vi "Examen 2 maquina de estados.vi"() -> ()   [LabVIEW 2021]
panel:
  out "LED":bool
  out "PUERTA":bool
  in  "Reset":bool
  out "#cafe":dbl
  in  "MANTENIMIENTO":bool
  out "#dulces":dbl
  out "#cafe 2":dbl
  out "#colombian":dbl
  out "#coca":dbl
  out "#pastel":dbl
  out "#dorito":dbl
  in  "Verificar":string
  in  "Coca-cola":bool
  in  "stop":bool
  out "Display":string
  out "CAMBIO":dbl
  out "EFECTIVO":dbl
  in  "COMPRAR":bool
  in  "capuchino":bool
  in  "coffe":bool
  in  "snacks Doritos":bool
  in  "Colombiana":bool
  in  "Candies":bool
  in  "pastel":bool
  in  "10":bool
  in  "20":bool
  # "MONEDAS"
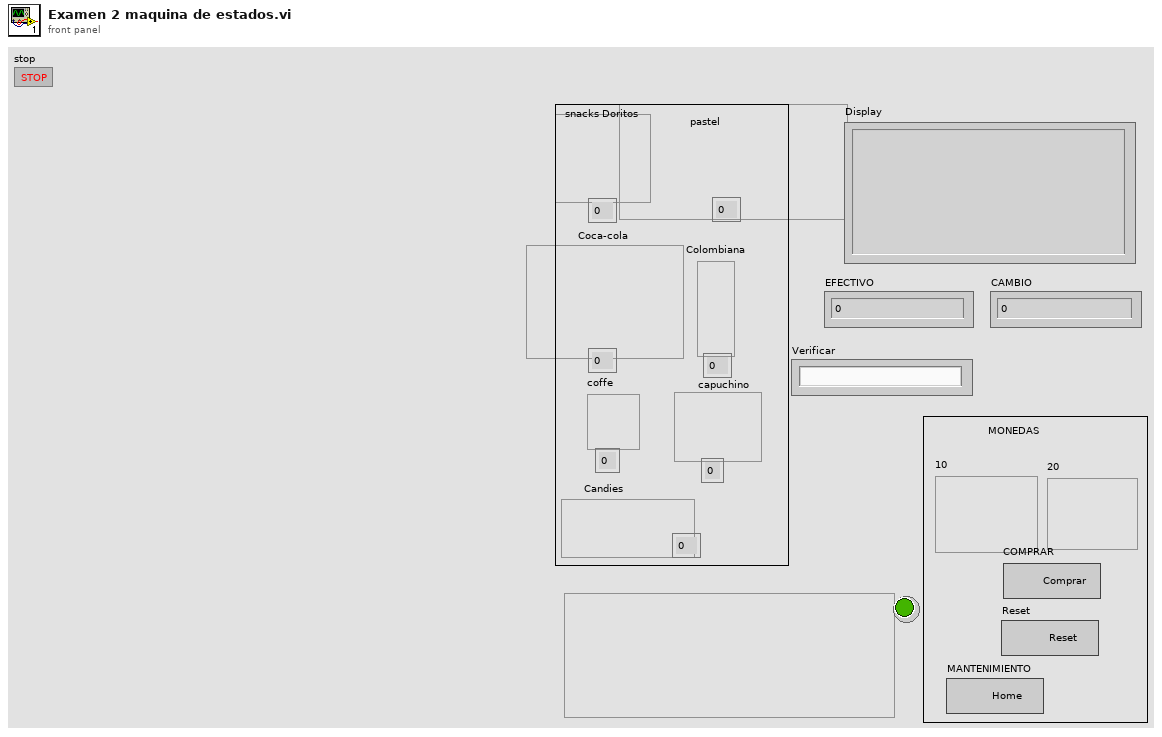
[diagram p1: front panel]
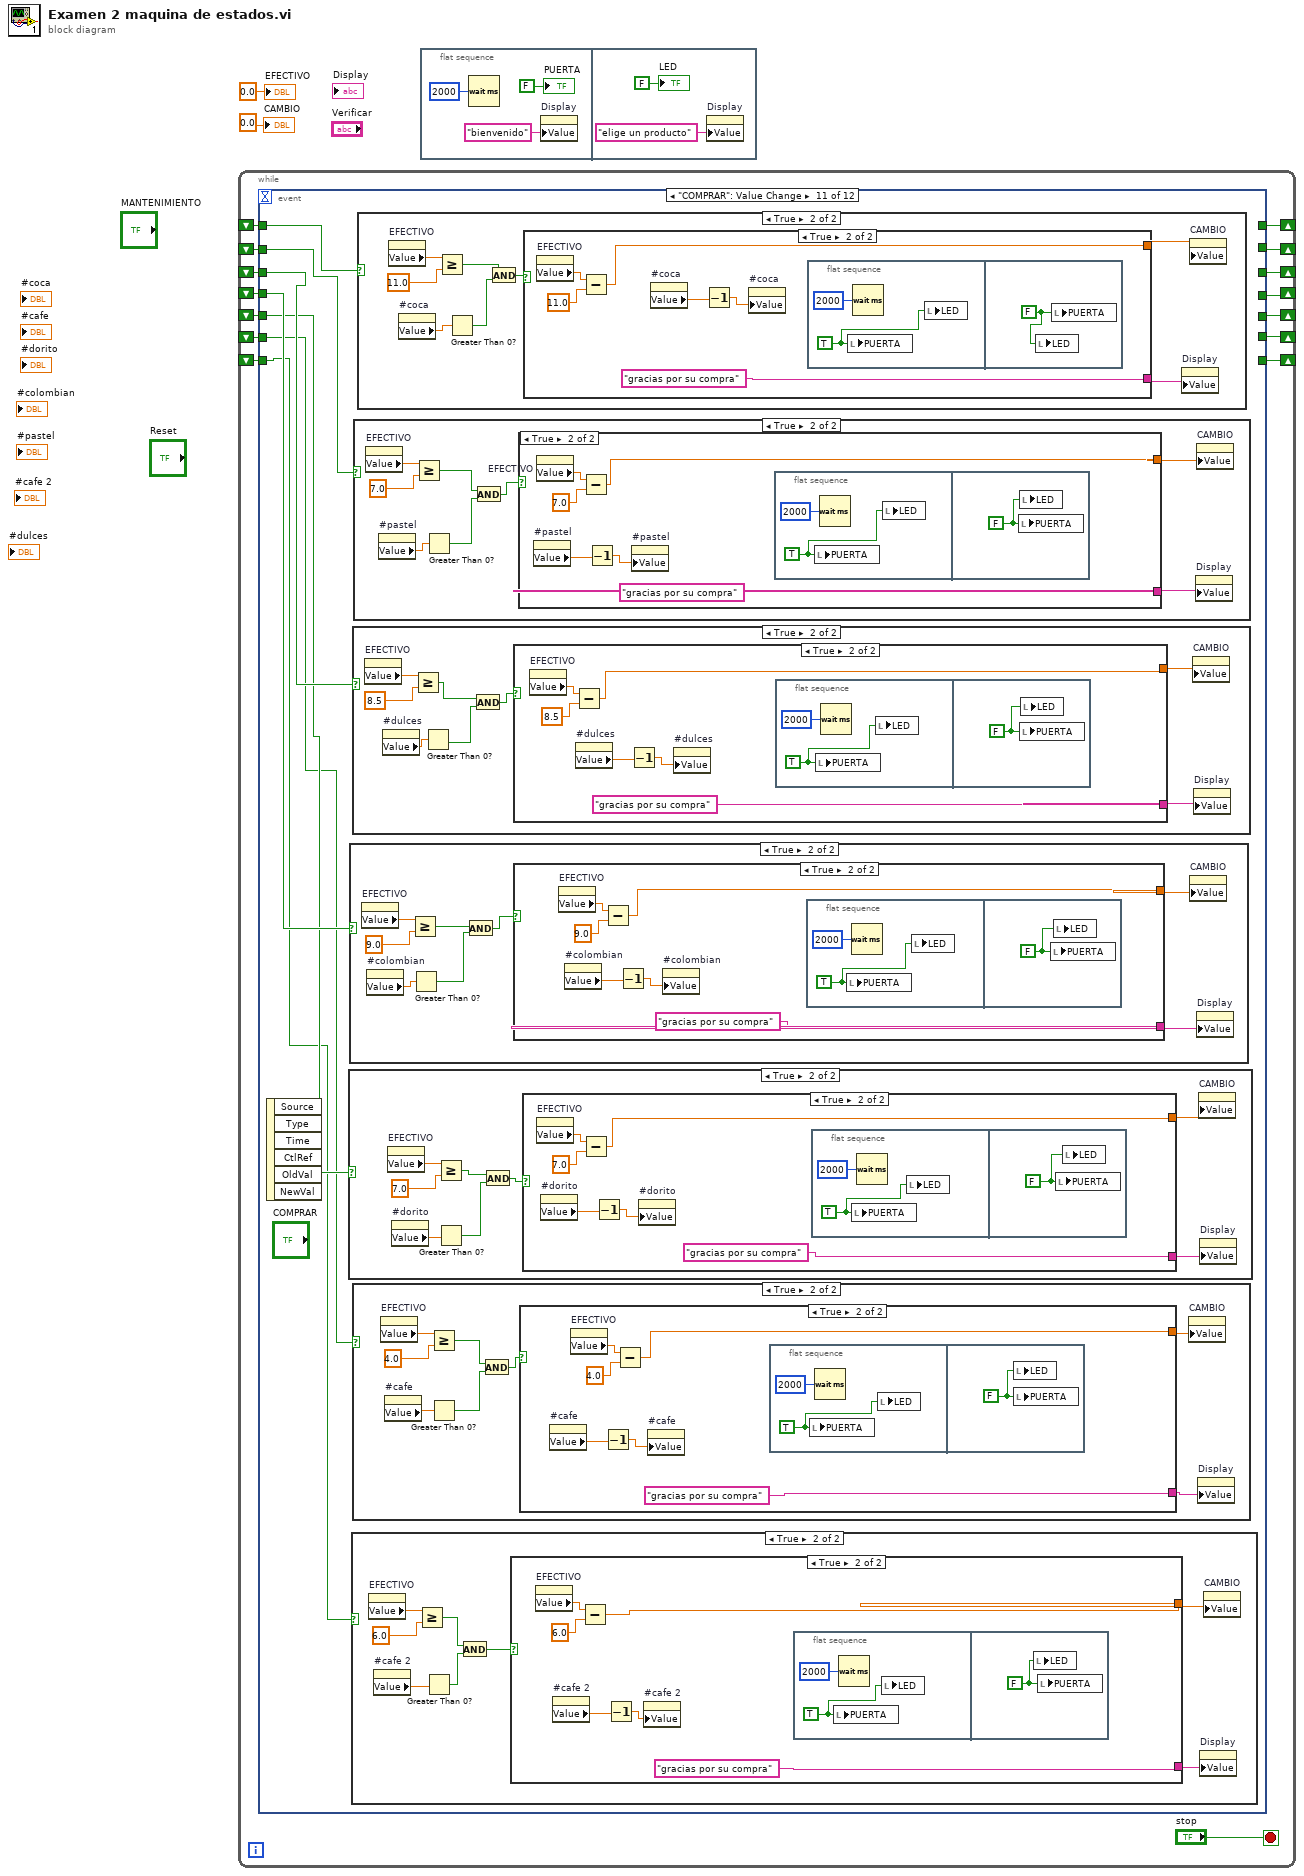
[diagram p0: block diagram]
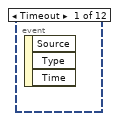
[diagram p2: hidden frame]
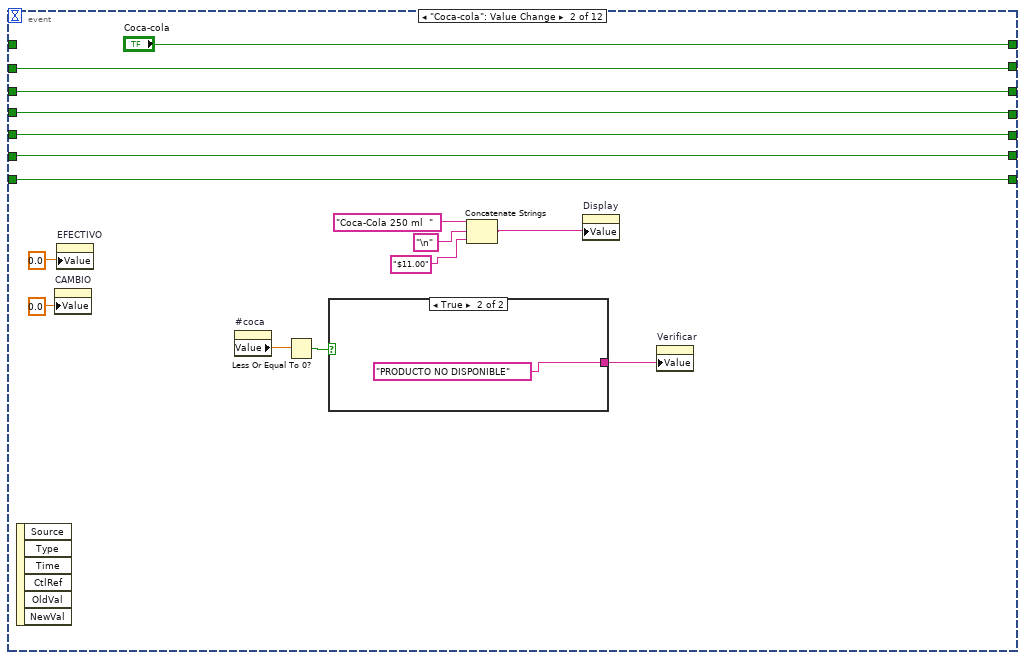
[diagram p3: hidden frame]
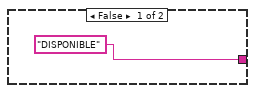
[diagram p4: hidden frame]
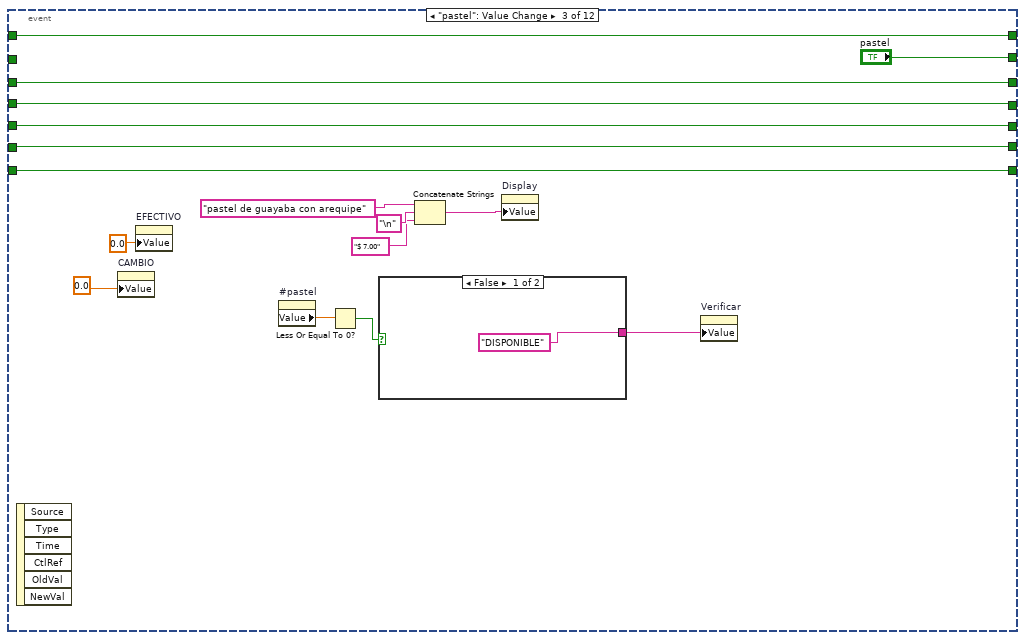
[diagram p5: hidden frame]
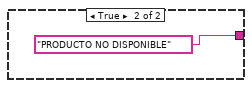
[diagram p6: hidden frame]
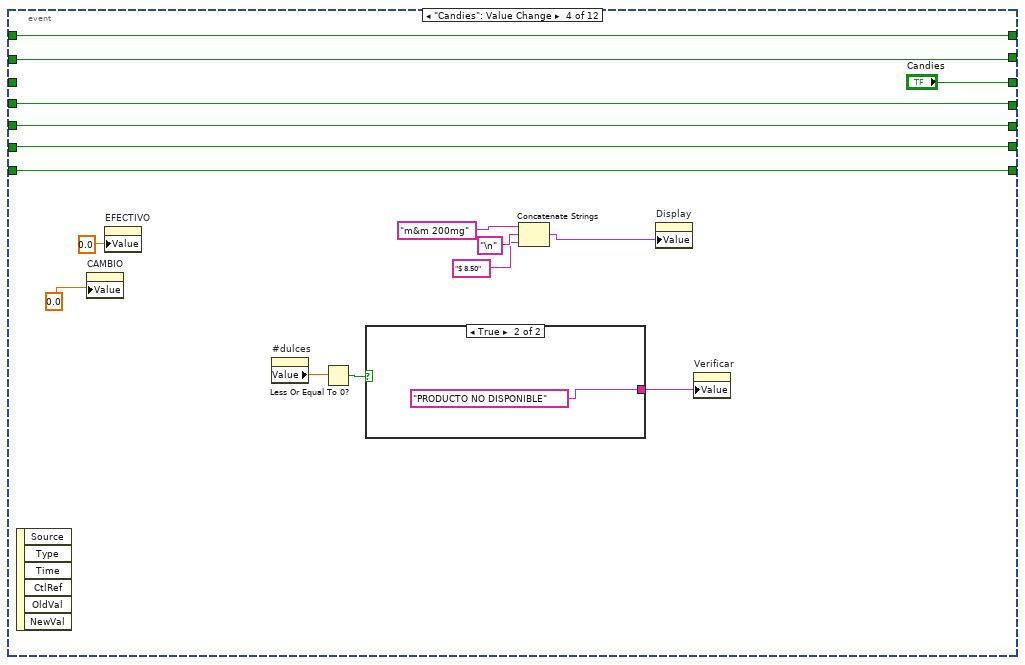
[diagram p7: hidden frame]
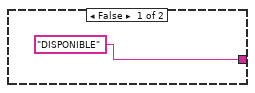
[diagram p8: hidden frame]
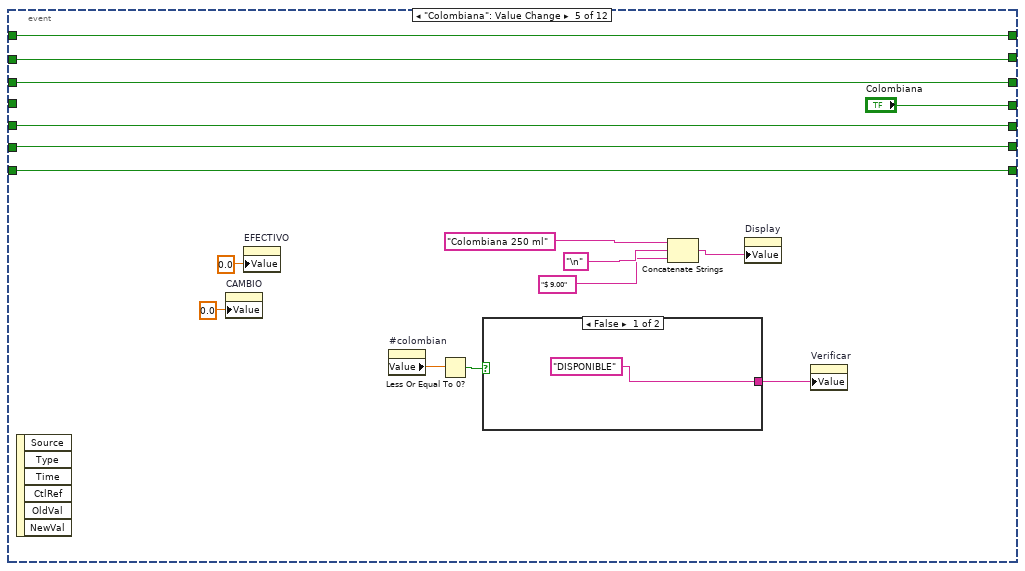
[diagram p9: hidden frame]
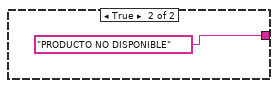
[diagram p10: hidden frame]
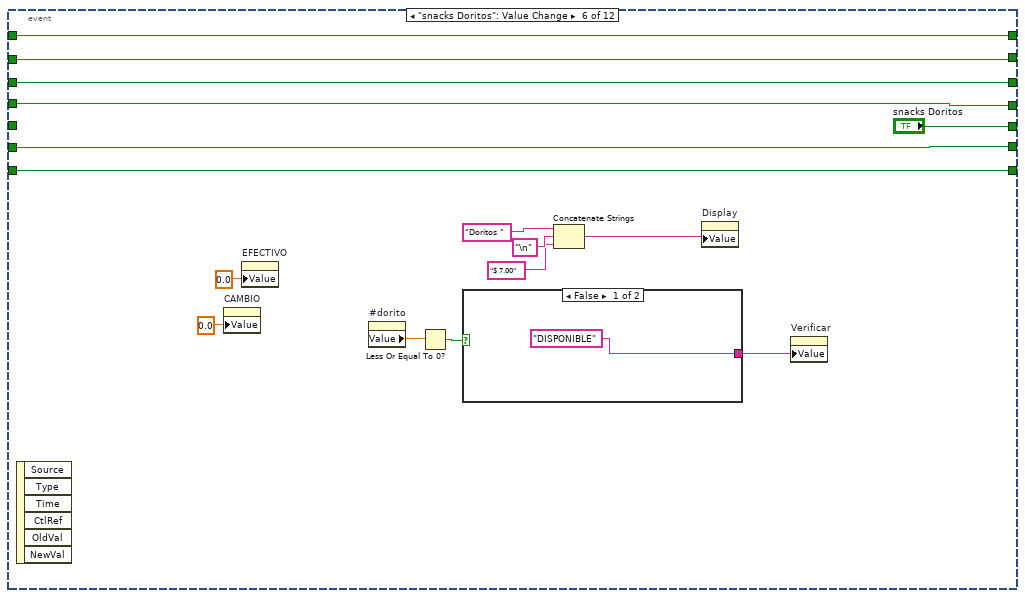
[diagram p11: hidden frame]
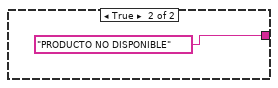
[diagram p12: hidden frame]
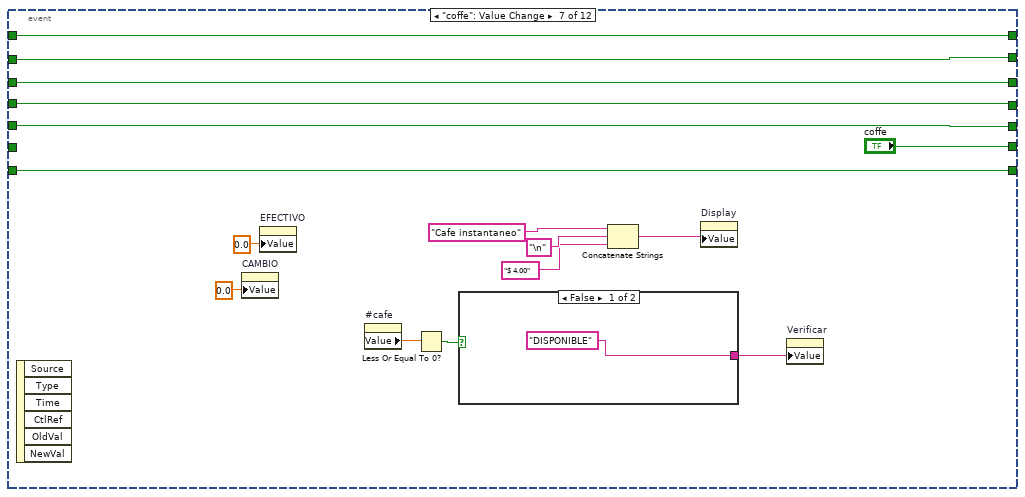
[diagram p13: hidden frame]
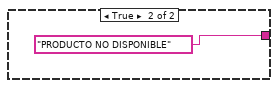
[diagram p14: hidden frame]
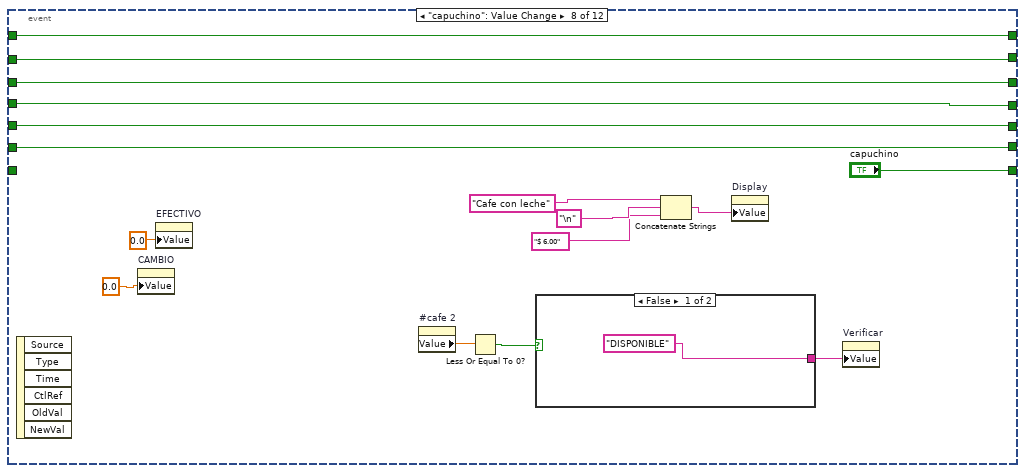
[diagram p15: hidden frame]
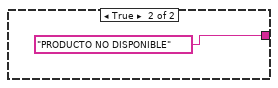
[diagram p16: hidden frame]
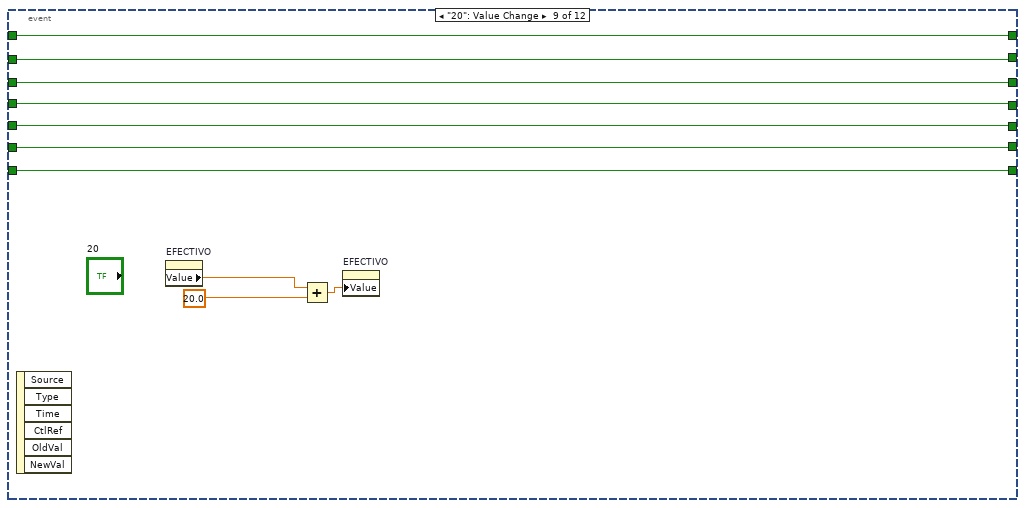
[diagram p17: hidden frame]
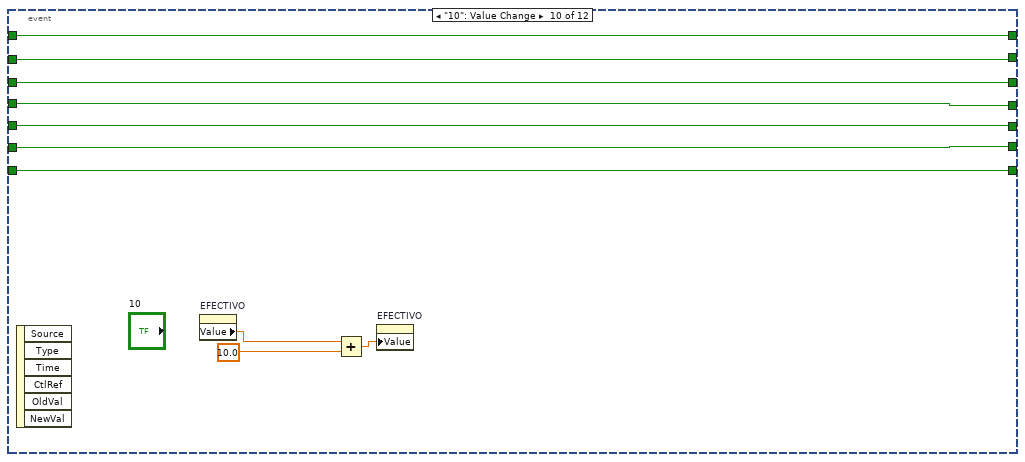
[diagram p18: hidden frame]
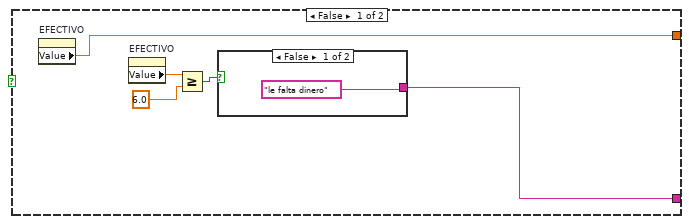
[diagram p20: hidden frame]
diagram:
  n1 = while {
    shift-right: [w16] -> _
    shift-left: _ -> [w15]
    shift-right: [w14] -> _
    shift-left: _ -> [w13]
    shift-right: [w12] -> _
    shift-left: _ -> [w11]
    shift-right: [w10] -> _
    shift-left: _ -> [w9]
    shift-right: [w8] -> _
    shift-left: _ -> [w7]
    shift-right: [w6] -> _
    shift-left: _ -> [w5]
    shift-right: [w4] -> _
    shift-left: _ -> [w3]
    stop <- "stop" stop-if-true
    n2 = event shown="[10] \"COMPRAR\": Value Change" {
      selector: _ -> [_ _ _ _ _ _ _ _ _ _ _ _]
      dyn-events: _ -> [_ _ _ _ _ _ _ _ _ _ _ _]
      timeout: _ -> [_ _ _ _ _ _ _ _ _ _ _ _]
      tunnel: [_ "Coca-cola" w51 w69 w87 w105 w123 w141 w150 w160 _ _] -> w16
      tunnel: w15 -> [_ _ w51 w69 w87 w105 w123 w141 w150 w160 w170 _]
      tunnel: [_ w30 "pastel" w66 w84 w102 w120 w138 w149 w159 _ _] -> w14
      tunnel: w13 -> [_ w30 _ w66 w84 w102 w120 w138 w149 w159 w169 _]
      tunnel: [_ w29 w47 "Candies" w83 w101 w119 w137 w148 w158 _ _] -> w12
      tunnel: w11 -> [_ w29 w47 _ w83 w101 w119 w137 w148 w158 w168 _]
      tunnel: [_ w28 w46 w64 "Colombiana" w100 w118 w136 w147 w157 _ _] -> w10
      tunnel: w9 -> [_ w28 w46 w64 _ w100 w118 w136 w147 w157 w167 _]
      tunnel: [_ w27 w45 w63 w81 "snacks Doritos" w117 w135 w146 w156 _ _] -> w8
      tunnel: w7 -> [_ w27 w45 w63 w81 _ w117 w135 w146 w156 w166 _]
      tunnel: [_ w26 w44 w62 w80 w98 "coffe" w134 w145 w155 _ _] -> w6
      tunnel: w5 -> [_ w26 w44 w62 w80 w98 _ w134 w145 w155 w165 _]
      tunnel: [_ w25 w43 w61 w79 w97 w115 "capuchino" w144 w154 _ _] -> w4
      tunnel: w3 -> [_ w25 w43 w61 w79 w97 w115 _ w144 w154 w164 _]
      event Timeout {
        n3 = event-data() -> ()  [unwired: 1 in, 3 out]
      }
      event "Coca-cola": Value Change {
        n4 = event-data() -> ()  [unwired: 1 in, 6 out]
        n5 = property on="CAMBIO" class="DigNum (strict)"("Value"=0.0 ("CAMBIO")) -> ()  [unwired: 2 in, 2 out]
        n6 = property on="EFECTIVO" class="DigNum (strict)"("Value"=0.0 ("EFECTIVO")) -> ()  [unwired: 2 in, 2 out]
        n7 = property on="#coca" class="DigNum (strict)"() -> ("Value"=w20:dbl)  [unwired: 2 in, 2 out]
        n8 = Less Or Equal To 0?(x=w20) -> (x <= 0?=w19:bool)
        n9 = case shown="True" w19 {
          tunnel: ["DISPONIBLE" "PRODUCTO NO DISPONIBLE"] -> w18
          frame False {
          }
          frame True {
          }
        }
        n10 = Concatenate Strings("Coca-Cola 250 ml  " ("Display"), "\n" ("string"), "$11.00" ("string")) -> (w21:string)
        n11 = property on="Display" class="Str"("Value"=w21) -> ()  [unwired: 2 in, 2 out]
        n12 = property on="Verificar" class="Str"("Value"=w18) -> ()  [unwired: 2 in, 2 out]
      }
      event "pastel": Value Change {
        n13 = event-data() -> ()  [unwired: 1 in, 6 out]
        n14 = property on="CAMBIO" class="DigNum (strict)"("Value"=0.0 ("CAMBIO")) -> ()  [unwired: 2 in, 2 out]
        n15 = property on="EFECTIVO" class="DigNum (strict)"("Value"=0.0 ("EFECTIVO")) -> ()  [unwired: 2 in, 2 out]
        n16 = property on="#pastel" class="DigNum (strict)"() -> ("Value"=w38:dbl)  [unwired: 2 in, 2 out]
        n17 = Less Or Equal To 0?(x=w38) -> (x <= 0?=w37:bool)
        n18 = case shown="False" w37 {
          tunnel: ["DISPONIBLE" "PRODUCTO NO DISPONIBLE"] -> w36
          frame False {
          }
          frame True {
          }
        }
        n19 = Concatenate Strings("pastel de guayaba con arequipe" ("Display"), "\n" ("string"), "$ 7.00" ("string")) -> (w39:string)
        n20 = property on="Display" class="Str"("Value"=w39) -> ()  [unwired: 2 in, 2 out]
        n21 = property on="Verificar" class="Str"("Value"=w36) -> ()  [unwired: 2 in, 2 out]
      }
      event "Candies": Value Change {
        n22 = event-data() -> ()  [unwired: 1 in, 6 out]
        n23 = property on="CAMBIO" class="DigNum (strict)"("Value"=0.0 ("CAMBIO")) -> ()  [unwired: 2 in, 2 out]
        n24 = property on="EFECTIVO" class="DigNum (strict)"("Value"=0.0 ("EFECTIVO")) -> ()  [unwired: 2 in, 2 out]
        n25 = property on="#dulces" class="DigNum (strict)"() -> ("Value"=w56:dbl)  [unwired: 2 in, 2 out]
        n26 = Less Or Equal To 0?(x=w56) -> (x <= 0?=w55:bool)
        n27 = case shown="True" w55 {
          tunnel: ["DISPONIBLE" "PRODUCTO NO DISPONIBLE"] -> w54
          frame False {
          }
          frame True {
          }
        }
        n28 = Concatenate Strings("m&m 200mg" ("Display"), "\n" ("string"), "$ 8.50" ("string")) -> (w57:string)
        n29 = property on="Display" class="Str"("Value"=w57) -> ()  [unwired: 2 in, 2 out]
        n30 = property on="Verificar" class="Str"("Value"=w54) -> ()  [unwired: 2 in, 2 out]
      }
      event "Colombiana": Value Change {
        n31 = event-data() -> ()  [unwired: 1 in, 6 out]
        n32 = property on="CAMBIO" class="DigNum (strict)"("Value"=0.0 ("CAMBIO")) -> ()  [unwired: 2 in, 2 out]
        n33 = property on="EFECTIVO" class="DigNum (strict)"("Value"=0.0 ("EFECTIVO")) -> ()  [unwired: 2 in, 2 out]
        n34 = property on="#colombian" class="DigNum (strict)"() -> ("Value"=w74:dbl)  [unwired: 2 in, 2 out]
        n35 = Less Or Equal To 0?(x=w74) -> (x <= 0?=w73:bool)
        n36 = case shown="False" w73 {
          tunnel: ["DISPONIBLE" "PRODUCTO NO DISPONIBLE"] -> w72
          frame False {
          }
          frame True {
          }
        }
        n37 = Concatenate Strings("Colombiana 250 ml" ("Display"), "\n" ("string"), "$ 9.00" ("string")) -> (w75:string)
        n38 = property on="Display" class="Str"("Value"=w75) -> ()  [unwired: 2 in, 2 out]
        n39 = property on="Verificar" class="Str"("Value"=w72) -> ()  [unwired: 2 in, 2 out]
      }
      event "snacks Doritos": Value Change {
        n40 = event-data() -> ()  [unwired: 1 in, 6 out]
        n41 = property on="CAMBIO" class="DigNum (strict)"("Value"=0.0 ("CAMBIO")) -> ()  [unwired: 2 in, 2 out]
        n42 = property on="EFECTIVO" class="DigNum (strict)"("Value"=0.0 ("EFECTIVO")) -> ()  [unwired: 2 in, 2 out]
        n43 = property on="#dorito" class="DigNum (strict)"() -> ("Value"=w92:dbl)  [unwired: 2 in, 2 out]
        n44 = Less Or Equal To 0?(x=w92) -> (x <= 0?=w91:bool)
        n45 = case shown="False" w91 {
          tunnel: ["DISPONIBLE" "PRODUCTO NO DISPONIBLE"] -> w90
          frame False {
          }
          frame True {
          }
        }
        n46 = Concatenate Strings("Doritos " ("Display"), "\n" ("string"), "$ 7.00" ("string")) -> (w93:string)
        n47 = property on="Display" class="Str"("Value"=w93) -> ()  [unwired: 2 in, 2 out]
        n48 = property on="Verificar" class="Str"("Value"=w90) -> ()  [unwired: 2 in, 2 out]
      }
      event "coffe": Value Change {
        n49 = event-data() -> ()  [unwired: 1 in, 6 out]
        n50 = property on="CAMBIO" class="DigNum (strict)"("Value"=0.0 ("CAMBIO")) -> ()  [unwired: 2 in, 2 out]
        n51 = property on="EFECTIVO" class="DigNum (strict)"("Value"=0.0 ("EFECTIVO")) -> ()  [unwired: 2 in, 2 out]
        n52 = property on="#cafe" class="DigNum (strict)"() -> ("Value"=w110:dbl)  [unwired: 2 in, 2 out]
        n53 = Less Or Equal To 0?(x=w110) -> (x <= 0?=w109:bool)
        n54 = case shown="False" w109 {
          tunnel: ["DISPONIBLE" "PRODUCTO NO DISPONIBLE"] -> w108
          frame False {
          }
          frame True {
          }
        }
        n55 = Concatenate Strings("Cafe instantaneo" ("Display"), "\n" ("string"), "$ 4.00" ("string")) -> (w111:string)
        n56 = property on="Display" class="Str"("Value"=w111) -> ()  [unwired: 2 in, 2 out]
        n57 = property on="Verificar" class="Str"("Value"=w108) -> ()  [unwired: 2 in, 2 out]
      }
      event "capuchino": Value Change {
        n58 = event-data() -> ()  [unwired: 1 in, 6 out]
        n59 = property on="CAMBIO" class="DigNum (strict)"("Value"=0.0 ("CAMBIO")) -> ()  [unwired: 2 in, 2 out]
        n60 = property on="EFECTIVO" class="DigNum (strict)"("Value"=0.0 ("EFECTIVO")) -> ()  [unwired: 2 in, 2 out]
        n61 = property on="#cafe 2" class="DigNum (strict)"() -> ("Value"=w128:dbl)  [unwired: 2 in, 2 out]
        n62 = Less Or Equal To 0?(x=w128) -> (x <= 0?=w127:bool)
        n63 = case shown="False" w127 {
          tunnel: ["DISPONIBLE" "PRODUCTO NO DISPONIBLE"] -> w126
          frame False {
          }
          frame True {
          }
        }
        n64 = Concatenate Strings("Cafe con leche" ("Display"), "\n" ("string"), "$ 6.00" ("string")) -> (w129:string)
        n65 = property on="Display" class="Str"("Value"=w129) -> ()  [unwired: 2 in, 2 out]
        n66 = property on="Verificar" class="Str"("Value"=w126) -> ()  [unwired: 2 in, 2 out]
      }
      event "20": Value Change {
        n67 = event-data() -> ()  [unwired: 1 in, 6 out]
        n68 = property on="EFECTIVO" class="DigNum (strict)"() -> ("Value"=w153:dbl)  [unwired: 2 in, 2 out]
        n69 = Add(x=w153, y=20.0) -> (x+y=w151:dbl)
        n70 = property on="EFECTIVO" class="DigNum (strict)"("Value"=w151) -> ()  [unwired: 2 in, 2 out]
      }
      event "10": Value Change {
        n71 = event-data() -> ()  [unwired: 1 in, 6 out]
        n72 = property on="EFECTIVO" class="DigNum (strict)"() -> ("Value"=w163:dbl)  [unwired: 2 in, 2 out]
        n73 = Add(x=w163, y=10.0) -> (x+y=w161:dbl)
        n74 = property on="EFECTIVO" class="DigNum (strict)"("Value"=w161) -> ()  [unwired: 2 in, 2 out]
      }
      event "COMPRAR": Value Change {
        n75 = event-data() -> ()  [unwired: 1 in, 6 out]
        n76 = case shown="True" w166 {
          frame False {
          }
          frame True {
            n77 = property on="EFECTIVO" class="DigNum (strict)"() -> ("Value"=w226:dbl)  [unwired: 2 in, 2 out]
            n78 = property on="#dorito" class="DigNum (strict)"() -> ("Value"=w222:dbl)  [unwired: 2 in, 2 out]
            n79 = Greater Or Equal?(x=w226, y=7.0) -> (x >= y?=w221:bool)
            n80 = Greater Than 0?(x=w222) -> (x > 0?=w220:bool)
            n81 = And(x=w221, y=w220) -> (x .and. y?=w219:bool)
            n82 = case shown="True" w219 {
              tunnel: [w231 w239] -> w224
              tunnel: [w227 "gracias por su compra" ("Display")] -> w223
              frame False {
                n83 = property on="EFECTIVO" class="DigNum (strict)"() -> ("Value"=w231:dbl)  [unwired: 2 in, 2 out]
                n84 = property on="EFECTIVO" class="DigNum (strict)"() -> ("Value"=w230:dbl)  [unwired: 2 in, 2 out]
                n85 = Greater Or Equal?(x=w230, y=7.0) -> (x >= y?=w228:bool)
                n86 = case shown="False" w228 {
                  tunnel: ["le falta dinero" ("Display") "PRODUCTO NO DISPONIBLE"] -> w227
                  frame False {
                  }
                  frame True {
                  }
                }
              }
              frame True {
                n87 = property on="EFECTIVO" class="DigNum (strict)"() -> ("Value"=w236:dbl)  [unwired: 2 in, 2 out]
                n88 = property on="#dorito" class="DigNum (strict)"() -> ("Value"=w234:dbl)  [unwired: 2 in, 2 out]
                n89 = Subtract(x=w236, y=7.0) -> (x-y=w239:dbl)
                n90 = Decrement(x=w234) -> (x-1=w235:dbl)
                n91 = property on="#dorito" class="DigNum (strict)"("Value"=w235) -> ()  [unwired: 2 in, 2 out]
                n92 = flat-sequence {
                  frame #0 {
                    w240 = TRUE ("PUERTA")
                    n93 = local write "PUERTA"(w240) -> ()
                    n94 = Wait (ms)(milliseconds to wait=u32 2000) -> ()  [unwired: 1 out]
                    n95 = local write "LED"(w240) -> ()
                  }
                  frame #1 {
                    w242 = FALSE ("PUERTA")
                    n96 = local write "PUERTA"(w242) -> ()
                    n97 = local write "LED"(w242) -> ()
                  }
                }
              }
            }
            n98 = property on="CAMBIO" class="DigNum (strict)"("Value"=w224) -> ()  [unwired: 2 in, 2 out]
            n99 = property on="Display" class="Str"("Value"=w223) -> ()  [unwired: 2 in, 2 out]
          }
        }
        n100 = case shown="True" w167 {
          frame False {
          }
          frame True {
            n101 = property on="EFECTIVO" class="DigNum (strict)"() -> ("Value"=w250:dbl)  [unwired: 2 in, 2 out]
            n102 = property on="#colombian" class="DigNum (strict)"() -> ("Value"=w246:dbl)  [unwired: 2 in, 2 out]
            n103 = Greater Or Equal?(x=w250, y=9.0) -> (x >= y?=w245:bool)
            n104 = Greater Than 0?(x=w246) -> (x > 0?=w244:bool)
            n105 = And(x=w245, y=w244) -> (x .and. y?=w243:bool)
            n106 = case shown="True" w243 {
              tunnel: [w255 w263] -> w248
              tunnel: [w251 "gracias por su compra" ("Display")] -> w247
              frame False {
                n107 = property on="EFECTIVO" class="DigNum (strict)"() -> ("Value"=w255:dbl)  [unwired: 2 in, 2 out]
                n108 = property on="EFECTIVO" class="DigNum (strict)"() -> ("Value"=w252:dbl)  [unwired: 2 in, 2 out]
                n109 = Greater Or Equal?(x=w252, y=9.0) -> (x >= y?=w254:bool)
                n110 = case shown="False" w254 {
                  tunnel: ["le falta dinero" ("Display") "PRODUCTO NO DISPONIBLE"] -> w251
                  frame False {
                  }
                  frame True {
                  }
                }
              }
              frame True {
                n111 = property on="EFECTIVO" class="DigNum (strict)"() -> ("Value"=w260:dbl)  [unwired: 2 in, 2 out]
                n112 = property on="#colombian" class="DigNum (strict)"() -> ("Value"=w259:dbl)  [unwired: 2 in, 2 out]
                n113 = Subtract(x=w260, y=9.0) -> (x-y=w263:dbl)
                n114 = Decrement(x=w259) -> (x-1=w258:dbl)
                n115 = property on="#colombian" class="DigNum (strict)"("Value"=w258) -> ()  [unwired: 2 in, 2 out]
                n116 = flat-sequence {
                  frame #0 {
                    w264 = TRUE ("PUERTA")
                    n117 = local write "PUERTA"(w264) -> ()
                    n118 = Wait (ms)(milliseconds to wait=u32 2000) -> ()  [unwired: 1 out]
                    n119 = local write "LED"(w264) -> ()
                  }
                  frame #1 {
                    w266 = FALSE ("PUERTA")
                    n120 = local write "PUERTA"(w266) -> ()
                    n121 = local write "LED"(w266) -> ()
                  }
                }
              }
            }
            n122 = property on="CAMBIO" class="DigNum (strict)"("Value"=w248) -> ()  [unwired: 2 in, 2 out]
            n123 = property on="Display" class="Str"("Value"=w247) -> ()  [unwired: 2 in, 2 out]
          }
        }
        n124 = case shown="True" w164 {
          frame False {
          }
          frame True {
            n125 = property on="EFECTIVO" class="DigNum (strict)"() -> ("Value"=w178:dbl)  [unwired: 2 in, 2 out]
            n126 = property on="#cafe 2" class="DigNum (strict)"() -> ("Value"=w174:dbl)  [unwired: 2 in, 2 out]
            n127 = Greater Or Equal?(x=w178, y=6.0) -> (x >= y?=w172:bool)
            n128 = Greater Than 0?(x=w174) -> (x > 0?=w171:bool)
            n129 = And(x=w172, y=w171) -> (x .and. y?=w173:bool)
            n130 = case shown="True" w173 {
              tunnel: [w183 w191] -> w176
              tunnel: [w179 "gracias por su compra" ("Display")] -> w175
              frame False {
                n131 = property on="EFECTIVO" class="DigNum (strict)"() -> ("Value"=w183:dbl)  [unwired: 2 in, 2 out]
                n132 = property on="EFECTIVO" class="DigNum (strict)"() -> ("Value"=w182:dbl)  [unwired: 2 in, 2 out]
                n133 = Greater Or Equal?(x=w182, y=6.0) -> (x >= y?=w180:bool)
                n134 = case shown="False" w180 {
                  tunnel: ["le falta dinero" ("Display") "PRODUCTO NO DISPONIBLE"] -> w179
                  frame False {
                  }
                  frame True {
                  }
                }
              }
              frame True {
                n135 = property on="EFECTIVO" class="DigNum (strict)"() -> ("Value"=w188:dbl)  [unwired: 2 in, 2 out]
                n136 = property on="#cafe 2" class="DigNum (strict)"() -> ("Value"=w186:dbl)  [unwired: 2 in, 2 out]
                n137 = Subtract(x=w188, y=6.0) -> (x-y=w191:dbl)
                n138 = Decrement(x=w186) -> (x-1=w187:dbl)
                n139 = property on="#cafe 2" class="DigNum (strict)"("Value"=w187) -> ()  [unwired: 2 in, 2 out]
                n140 = flat-sequence {
                  frame #0 {
                    w192 = TRUE ("PUERTA")
                    n141 = local write "PUERTA"(w192) -> ()
                    n142 = Wait (ms)(milliseconds to wait=u32 2000) -> ()  [unwired: 1 out]
                    n143 = local write "LED"(w192) -> ()
                  }
                  frame #1 {
                    w194 = FALSE ("PUERTA")
                    n144 = local write "LED"(w194) -> ()
                    n145 = local write "PUERTA"(w194) -> ()
                  }
                }
              }
            }
            n146 = property on="Display" class="Str"("Value"=w175) -> ()  [unwired: 2 in, 2 out]
            n147 = property on="CAMBIO" class="DigNum (strict)"("Value"=w176) -> ()  [unwired: 2 in, 2 out]
          }
        }
        n148 = case shown="True" w168 {
          frame False {
          }
          frame True {
            n149 = property on="EFECTIVO" class="DigNum (strict)"() -> ("Value"=w274:dbl)  [unwired: 2 in, 2 out]
            n150 = property on="#dulces" class="DigNum (strict)"() -> ("Value"=w270:dbl)  [unwired: 2 in, 2 out]
            n151 = Greater Or Equal?(x=w274, y=8.5) -> (x >= y?=w268:bool)
            n152 = Greater Than 0?(x=w270) -> (x > 0?=w269:bool)
            n153 = And(x=w268, y=w269) -> (x .and. y?=w267:bool)
            n154 = case shown="True" w267 {
              tunnel: [w279 w287] -> w272
              tunnel: [w275 "gracias por su compra" ("Display")] -> w271
              frame False {
                n155 = property on="EFECTIVO" class="DigNum (strict)"() -> ("Value"=w279:dbl)  [unwired: 2 in, 2 out]
                n156 = property on="EFECTIVO" class="DigNum (strict)"() -> ("Value"=w278:dbl)  [unwired: 2 in, 2 out]
                n157 = Greater Or Equal?(x=w278, y=8.5) -> (x >= y?=w276:bool)
                n158 = case shown="True" w276 {
                  tunnel: ["le falta dinero" ("Display") "PRODUCTO NO DISPONIBLE"] -> w275
                  frame False {
                  }
                  frame True {
                  }
                }
              }
              frame True {
                n159 = property on="EFECTIVO" class="DigNum (strict)"() -> ("Value"=w284:dbl)  [unwired: 2 in, 2 out]
                n160 = Subtract(x=w284, y=8.5) -> (x-y=w287:dbl)
                n161 = property on="#dulces" class="DigNum (strict)"() -> ("Value"=w282:dbl)  [unwired: 2 in, 2 out]
                n162 = Decrement(x=w282) -> (x-1=w283:dbl)
                n163 = property on="#dulces" class="DigNum (strict)"("Value"=w283) -> ()  [unwired: 2 in, 2 out]
                n164 = flat-sequence {
                  frame #0 {
                    w288 = TRUE ("PUERTA")
                    n165 = local write "PUERTA"(w288) -> ()
                    n166 = Wait (ms)(milliseconds to wait=u32 2000) -> ()  [unwired: 1 out]
                    n167 = local write "LED"(w288) -> ()
                  }
                  frame #1 {
                    w290 = FALSE ("PUERTA")
                    n168 = local write "PUERTA"(w290) -> ()
                    n169 = local write "LED"(w290) -> ()
                  }
                }
              }
            }
            n170 = property on="CAMBIO" class="DigNum (strict)"("Value"=w272) -> ()  [unwired: 2 in, 2 out]
            n171 = property on="Display" class="Str"("Value"=w271) -> ()  [unwired: 2 in, 2 out]
          }
        }
        n172 = case shown="True" w165 {
          frame False {
          }
          frame True {
            n173 = property on="EFECTIVO" class="DigNum (strict)"() -> ("Value"=w202:dbl)  [unwired: 2 in, 2 out]
            n174 = property on="#cafe" class="DigNum (strict)"() -> ("Value"=w198:dbl)  [unwired: 2 in, 2 out]
            n175 = Greater Or Equal?(x=w202, y=4.0) -> (x >= y?=w196:bool)
            n176 = Greater Than 0?(x=w198) -> (x > 0?=w197:bool)
            n177 = And(x=w196, y=w197) -> (x .and. y?=w195:bool)
            n178 = case shown="True" w195 {
              tunnel: [w207 w213] -> w200
              tunnel: [w203 "gracias por su compra" ("Display")] -> w199
              frame False {
                n179 = property on="EFECTIVO" class="DigNum (strict)"() -> ("Value"=w207:dbl)  [unwired: 2 in, 2 out]
                n180 = property on="EFECTIVO" class="DigNum (strict)"() -> ("Value"=w204:dbl)  [unwired: 2 in, 2 out]
                n181 = Greater Or Equal?(x=w204, y=4.0) -> (x >= y?=w206:bool)
                n182 = case shown="True" w206 {
                  tunnel: ["le falta dinero" ("Display") "PRODUCTO NO DISPONIBLE"] -> w203
                  frame False {
                  }
                  frame True {
                  }
                }
              }
              frame True {
                n183 = property on="#cafe" class="DigNum (strict)"() -> ("Value"=w211:dbl)  [unwired: 2 in, 2 out]
                n184 = property on="EFECTIVO" class="DigNum (strict)"() -> ("Value"=w214:dbl)  [unwired: 2 in, 2 out]
                n185 = Decrement(x=w211) -> (x-1=w210:dbl)
                n186 = Subtract(x=w214, y=4.0) -> (x-y=w213:dbl)
                n187 = property on="#cafe" class="DigNum (strict)"("Value"=w210) -> ()  [unwired: 2 in, 2 out]
                n188 = flat-sequence {
                  frame #0 {
                    w216 = TRUE ("PUERTA")
                    n189 = local write "PUERTA"(w216) -> ()
                    n190 = Wait (ms)(milliseconds to wait=u32 2000) -> ()  [unwired: 1 out]
                    n191 = local write "LED"(w216) -> ()
                  }
                  frame #1 {
                    w218 = FALSE ("PUERTA")
                    n192 = local write "LED"(w218) -> ()
                    n193 = local write "PUERTA"(w218) -> ()
                  }
                }
              }
            }
            n194 = property on="CAMBIO" class="DigNum (strict)"("Value"=w200) -> ()  [unwired: 2 in, 2 out]
            n195 = property on="Display" class="Str"("Value"=w199) -> ()  [unwired: 2 in, 2 out]
          }
        }
        n196 = case shown="True" w169 {
          frame False {
          }
          frame True {
            n197 = property on="EFECTIVO" class="DigNum (strict)"() -> ("Value"=w298:dbl)  [unwired: 2 in, 2 out]
            n198 = property on="#pastel" class="DigNum (strict)"() -> ("Value"=w294:dbl)  [unwired: 2 in, 2 out]
            n199 = Greater Or Equal?(x=w298, y=7.0) -> (x >= y?=w292:bool)
            n200 = Greater Than 0?(x=w294) -> (x > 0?=w291:bool)
            n201 = And(x=w292, y=w291) -> (x .and. y?=w293:bool)
            n202 = case shown="True" w293 {
              tunnel: [w303 w311] -> w296
              tunnel: [w299 "gracias por su compra" ("Display")] -> w295
              frame False {
                n203 = property on="EFECTIVO" class="DigNum (strict)"() -> ("Value"=w303:dbl)  [unwired: 2 in, 2 out]
                n204 = property on="EFECTIVO" class="DigNum (strict)"() -> ("Value"=w300:dbl)  [unwired: 2 in, 2 out]
                n205 = Greater Or Equal?(x=w300, y=7.0) -> (x >= y?=w302:bool)
                n206 = case shown="True" w302 {
                  tunnel: ["le falta dinero" ("Display") "PRODUCTO NO DISPONIBLE"] -> w299
                  frame False {
                  }
                  frame True {
                  }
                }
              }
              frame True {
                n207 = property on="#pastel" class="DigNum (strict)"() -> ("Value"=w307:dbl)  [unwired: 2 in, 2 out]
                n208 = property on="EFECTIVO" class="DigNum (strict)"() -> ("Value"=w308:dbl)  [unwired: 2 in, 2 out]
                n209 = Subtract(x=w308, y=7.0) -> (x-y=w311:dbl)
                n210 = Decrement(x=w307) -> (x-1=w306:dbl)
                n211 = property on="#pastel" class="DigNum (strict)"("Value"=w306) -> ()  [unwired: 2 in, 2 out]
                n212 = flat-sequence {
                  frame #0 {
                    w312 = TRUE ("PUERTA")
                    n213 = local write "PUERTA"(w312) -> ()
                    n214 = Wait (ms)(milliseconds to wait=u32 2000) -> ()  [unwired: 1 out]
                    n215 = local write "LED"(w312) -> ()
                  }
                  frame #1 {
                    w314 = FALSE ("PUERTA")
                    n216 = local write "PUERTA"(w314) -> ()
                    n217 = local write "LED"(w314) -> ()
                  }
                }
              }
            }
            n218 = property on="Display" class="Str"("Value"=w295) -> ()  [unwired: 2 in, 2 out]
            n219 = property on="CAMBIO" class="DigNum (strict)"("Value"=w296) -> ()  [unwired: 2 in, 2 out]
          }
        }
        n220 = case shown="True" w170 {
          frame False {
          }
          frame True {
            n221 = property on="EFECTIVO" class="DigNum (strict)"() -> ("Value"=w322:dbl)  [unwired: 2 in, 2 out]
            n222 = property on="#coca" class="DigNum (strict)"() -> ("Value"=w317:dbl)  [unwired: 2 in, 2 out]
            n223 = Greater Or Equal?(x=w322, y=11.0) -> (x >= y?=w318:bool)
            n224 = Greater Than 0?(x=w317) -> (x > 0?=w316:bool)
            n225 = And(x=w318, y=w316) -> (x .and. y?=w315:bool)
            n226 = case shown="True" w315 {
              tunnel: [w327 w335] -> w320
              tunnel: [w323 "gracias por su compra" ("Display")] -> w319
              frame False {
                n227 = property on="EFECTIVO" class="DigNum (strict)"() -> ("Value"=w327:dbl)  [unwired: 2 in, 2 out]
                n228 = property on="EFECTIVO" class="DigNum (strict)"() -> ("Value"=w326:dbl)  [unwired: 2 in, 2 out]
                n229 = Greater Or Equal?(x=w326, y=11.0) -> (x >= y?=w324:bool)
                n230 = case shown="False" w324 {
                  tunnel: ["le falta dinero" ("Display") "PRODUCTO NO DISPONIBLE"] -> w323
                  frame False {
                  }
                  frame True {
                  }
                }
              }
              frame True {
                n231 = property on="EFECTIVO" class="DigNum (strict)"() -> ("Value"=w332:dbl)  [unwired: 2 in, 2 out]
                n232 = Subtract(x=w332, y=11.0) -> (x-y=w335:dbl)
                n233 = property on="#coca" class="DigNum (strict)"() -> ("Value"=w331:dbl)  [unwired: 2 in, 2 out]
                n234 = Decrement(x=w331) -> (x-1=w330:dbl)
                n235 = property on="#coca" class="DigNum (strict)"("Value"=w330) -> ()  [unwired: 2 in, 2 out]
                n236 = flat-sequence {
                  frame #0 {
                    w336 = TRUE ("PUERTA")
                    n237 = local write "PUERTA"(w336) -> ()
                    n238 = Wait (ms)(milliseconds to wait=u32 2000) -> ()  [unwired: 1 out]
                    n239 = local write "LED"(w336) -> ()
                  }
                  frame #1 {
                    w338 = FALSE ("PUERTA")
                    n240 = local write "LED"(w338) -> ()
                    n241 = local write "PUERTA"(w338) -> ()
                  }
                }
              }
            }
            n242 = property on="Display" class="Str"("Value"=w319) -> ()  [unwired: 2 in, 2 out]
            n243 = property on="CAMBIO" class="DigNum (strict)"("Value"=w320) -> ()  [unwired: 2 in, 2 out]
          }
        }
      }
      event "Reset": Value Change {
        n244 = event-data() -> ()  [unwired: 1 in, 6 out]
        n245 = property on="EFECTIVO" class="DigNum (strict)"("Value"=0.0 ("EFECTIVO")) -> ()  [unwired: 2 in, 2 out]
        n246 = property on="CAMBIO" class="DigNum (strict)"("Value"=0.0 ("CAMBIO")) -> ()  [unwired: 2 in, 2 out]
        n247 = property on="Display" class="Str"("Value"="bienvenido" ("Display")) -> ()  [unwired: 2 in, 2 out]
      }
    }
  }
  n248 = flat-sequence {
    frame #0 {
      n249 = Wait (ms)(milliseconds to wait=u32 2000) -> ()  [unwired: 1 out]
      n250 = property on="Display" class="Str"("Value"="bienvenido" ("Display")) -> ()  [unwired: 2 in, 2 out]
      "PUERTA" <- FALSE ("PUERTA")
    }
    frame #1 {
      n251 = property on="Display" class="Str"("Value"="elige un producto" ("Display")) -> ()  [unwired: 2 in, 2 out]
      "LED" <- FALSE
    }
  }
  "EFECTIVO" <- 0.0 ("EFECTIVO")
  "CAMBIO" <- 0.0 ("CAMBIO")
